vi "set pid array.vi"(8 "error in (no error)":errorcluster, 10 "Array":T2[](array[typedef]), 11 "Array in":T1) -> (0 "error out":errorcluster, 3 "Array out":T1)   [LabVIEW 2015, in "PID Module editor node.lvclass"]
uses:
  PID Module editor node.lvclass
  PID array reference.ctl
  PID array element.ctl
  module/configuration/PID Module configuration.lvclass
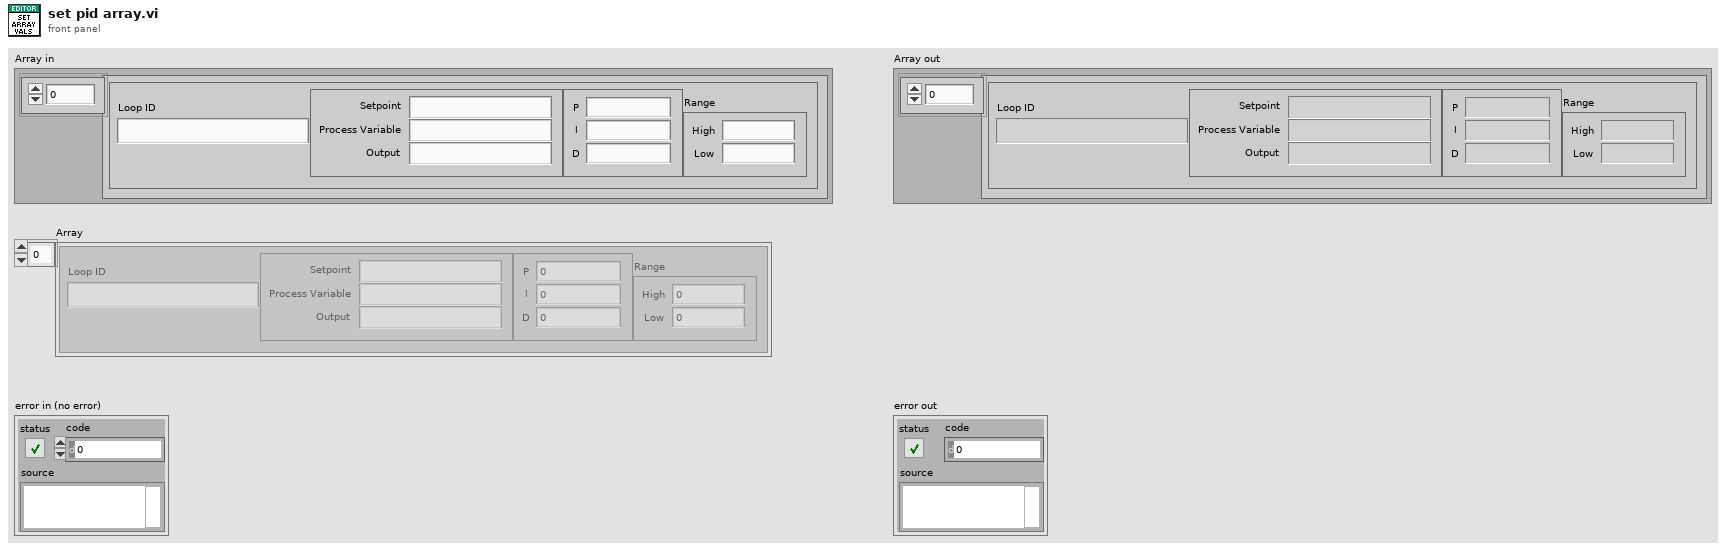
[diagram p1: front panel]
types:
  T1 = typedef "PID Module editor node.lvclass/PID array reference.ctl" = refnum<vi>
  T2 = typedef "PID Module configuration.lvclass/PID array element.ctl" = cluster{"Loop ID":string, "Tags":cluster{"Setpoint":string, "Process Variable":string, "Output":string}, "Gains":cluster{"P":dbl, "I":dbl, "D":dbl}, "Range":cluster{"High":dbl, "Low":dbl}}
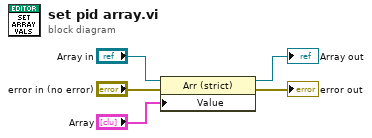
[diagram p0: block diagram]
diagram:
  n1 = property class="Arr (strict)"(reference="Array in", error in="error in (no error)", "Value"="Array") -> (reference out=→"Array out":T1, error out=→"error out":errorcluster)
